vi "advanced.filter.dialog.vi"(5 "filters events":refnum<user-event>, 7 "manager_daemon":refnum<class "manager_daemon.lvclass">, 8 "filter exit event":refnum<user-event>, 9 "filtered publisher ids":i32[](array[numeric]), 10 "map":T2, 11 "pub filter event":refnum<user-event>) -> ()   [LabVIEW 2024]
uses:
  comic_manager/manager_daemon/type_defs/PublisherMap--map.ctl
  comic_manager/manager_daemon/type_defs/PublisherData--cluster.ctl
  selection_dropdown/Typedefs/Selection Dropdown--cluster.ctl
  comic_manager/manager_daemon/manager_daemon.lvclass
  typedefs/filters--cluster.ctl
  selection_dropdown/selection_dropdown.lvclass/selection_dropdown.ctl
  selection_dropdown/selection_dropdown.lvclass
  <vilib>/addons/_JKI Toolkits/State Machine/_JKI_lib_State_Machine.llb/Select State(s)_err__jki_lib_state_machine.vi
  <vilib>/addons/_JKI Toolkits/State Machine/_JKI_lib_State_Machine.llb/Periodic Trigger__ogtk__JKI-SM__jki_lib_state_machine.vi
panel:
  in  "Apply Filters":enum32{"AND", "OR"}(radio)=enum."OR"
  in  "concept filter":T1
  in  "storyArc filter":T1
  in  "character filter":T1
  in  "team filter":T1
  in  "select none":bool
  in  "select all":bool
  in  "clear error":bool
  in  "Exit":bool
  out "error out":errorcluster
  in  "pub listbox":i32(listbox)
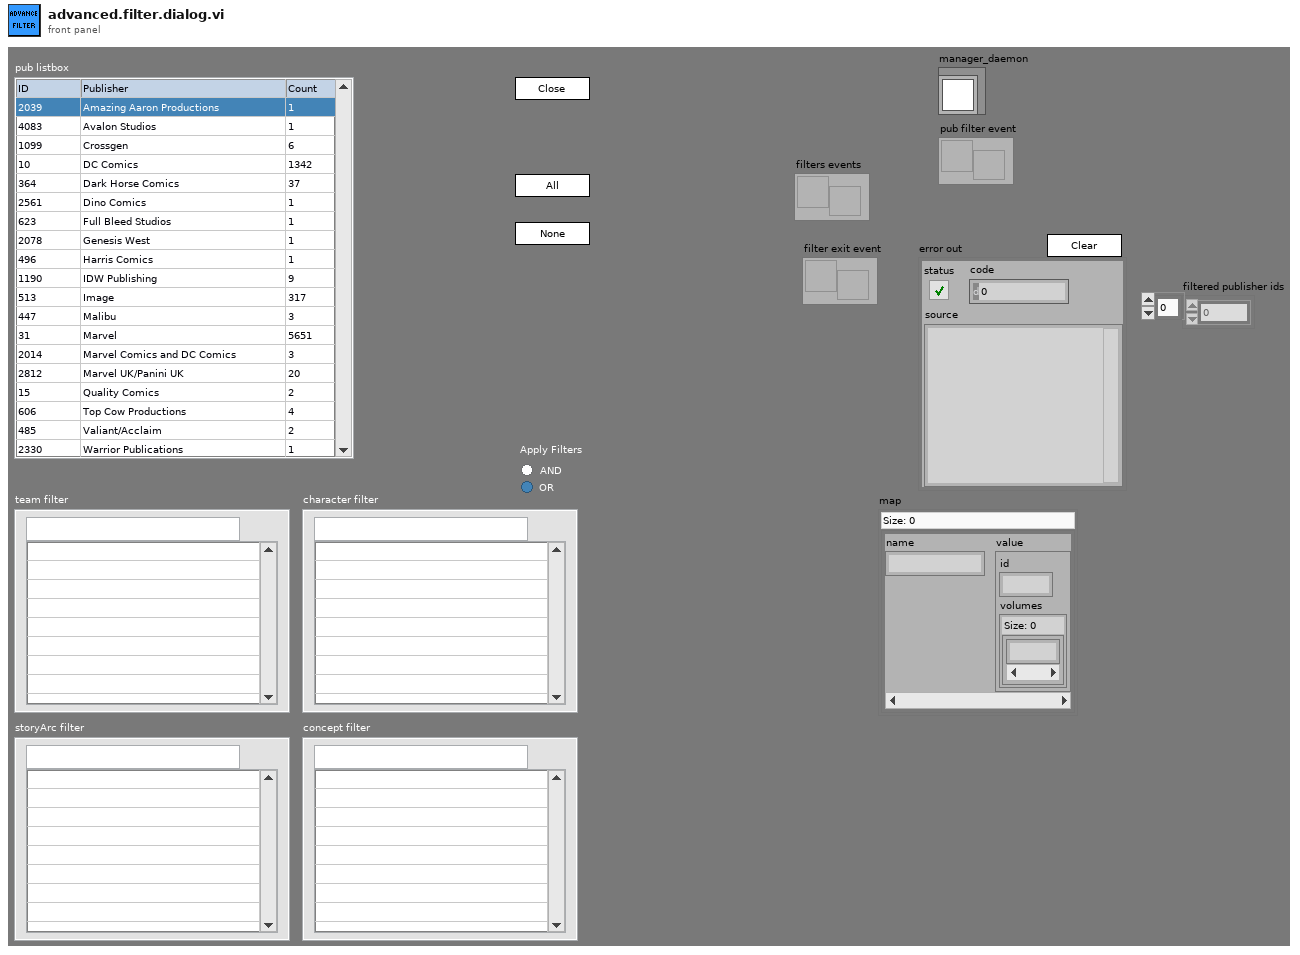
[diagram p1: front panel]
types:
  T1 = typedef "selection_dropdown.lvclass/Selection Dropdown--cluster.ctl" = cluster{"available":i32, "list":i32, "cancel":bool, "selection":string}
  T2 = typedef "manager_daemon.lvclass/PublisherMap--map.ctl" = map{string, T3}
  T3 = typedef "manager_daemon.lvclass/PublisherData--cluster.ctl" = cluster{"id":i32, "volumes":set{i32}}
  T4 = enum32{"Invalid", "Standard", "Closed", "Hidden", "Minimized", "Maximized"}
  T5 = enum32{"invalid app kind", "Development System", "Run Time System", "Student Edition", "Embedded LabVIEW", "Evaluation", "Custom"}
  T6 = typedef "filters--cluster.ctl" = cluster{"team filter":string[], "story filter":string[], "char filter":string[], "concept filter":string[], "Apply Filters":enum32{"AND", "OR"}}
  T7 = cluster{"Core":cluster{"Current VI Reference":refnum<vi>, "Close Panel on Exit?":bool}, "pub ids":i32[], "pub symbols":i32[], "pub filter event":refnum<user-event>, "filters":cluster{"team filter":refnum<class "selection_dropdown.lvclass">, "story filter":refnum<class "selection_dropdown.lvclass">, "char filter":refnum<class "selection_dropdown.lvclass">, "concept filter":refnum<class "selection_dropdown.lvclass">}, "manager_daemon":refnum<class "manager_daemon.lvclass">, "filters events":refnum<user-event>, "filter exit event":refnum<user-event>}
  T8 = cluster{"team filter":refnum<class "selection_dropdown.lvclass">, "story filter":refnum<class "selection_dropdown.lvclass">, "char filter":refnum<class "selection_dropdown.lvclass">, "concept filter":refnum<class "selection_dropdown.lvclass">}
  T9 = cluster{"Current VI Reference":refnum<vi>, "Close Panel on Exit?":bool}
  T10 = cluster{"team filter event":refnum<user-event>, "story filter event":refnum<user-event>, "char filter event":refnum<user-event>, "concept filter event":refnum<user-event>}
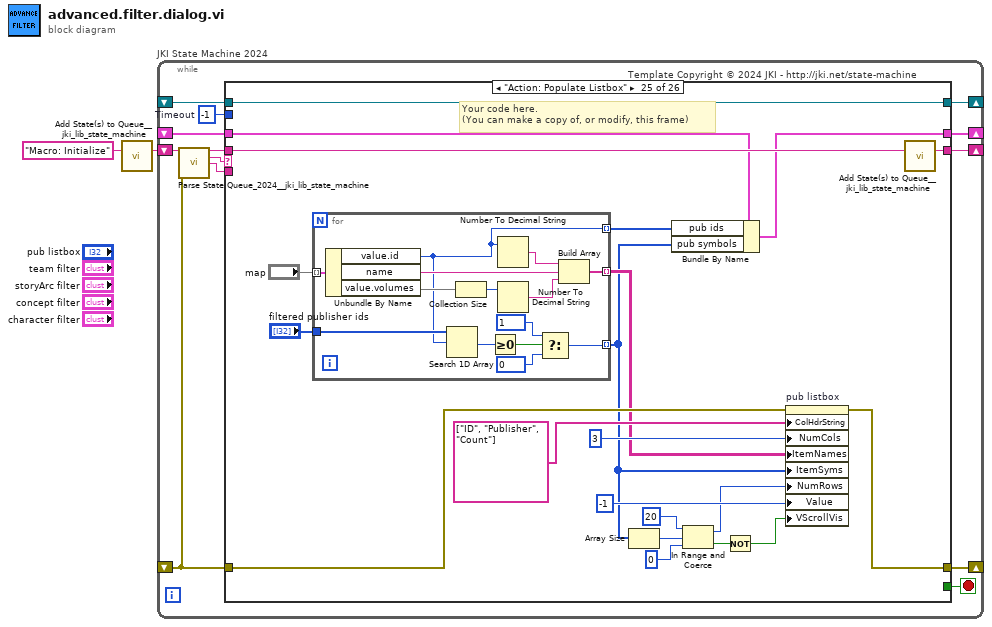
[diagram p0: block diagram]
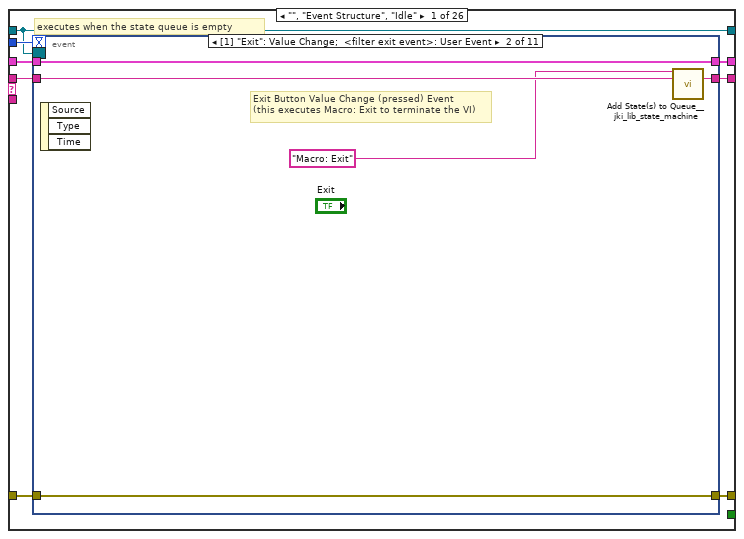
[diagram p2: hidden frame]
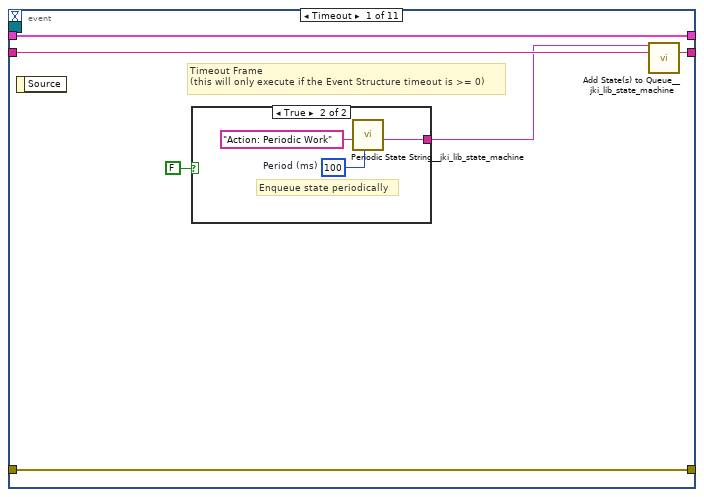
[diagram p3: hidden frame]
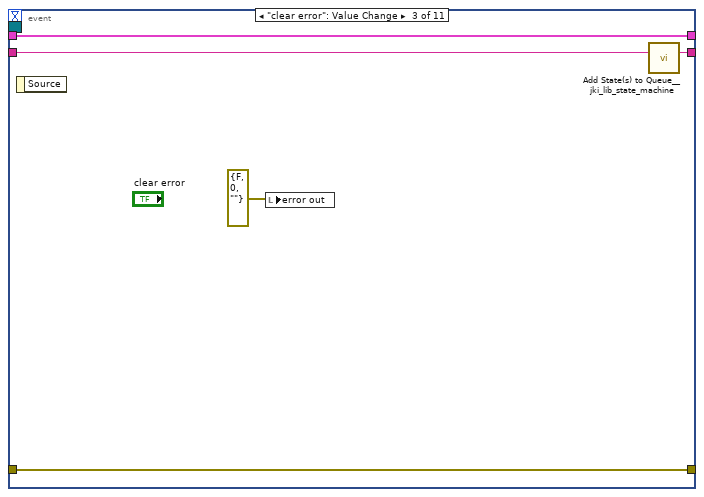
[diagram p5: hidden frame]
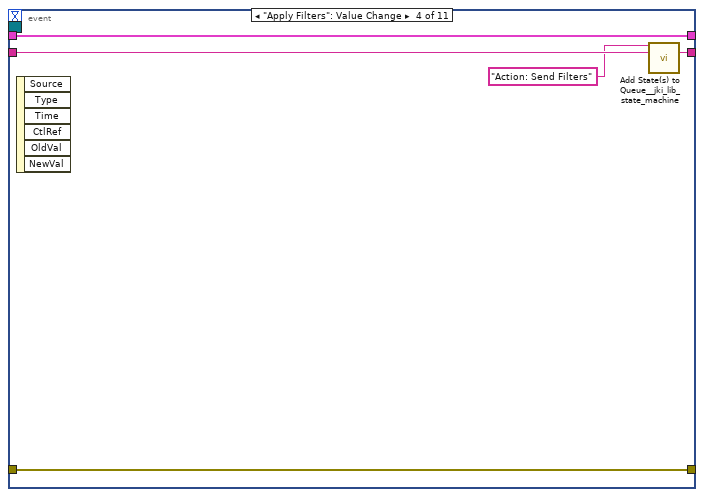
[diagram p6: hidden frame]
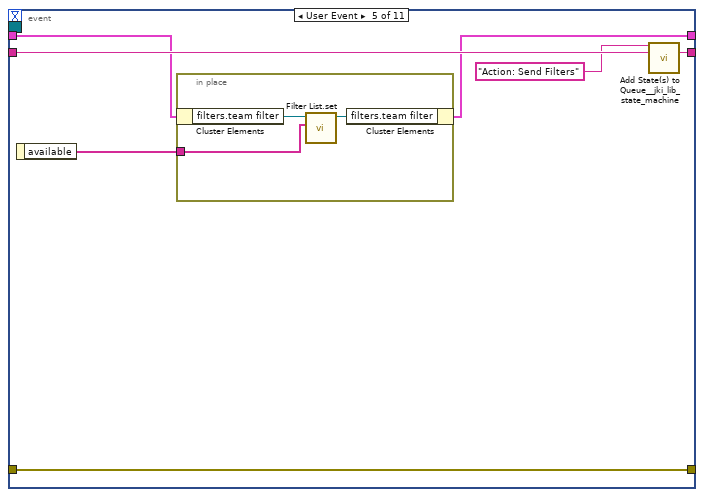
[diagram p7: hidden frame]
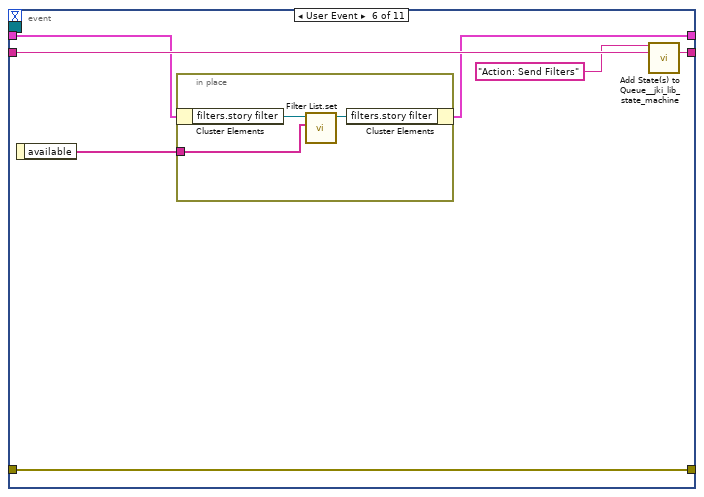
[diagram p8: hidden frame]
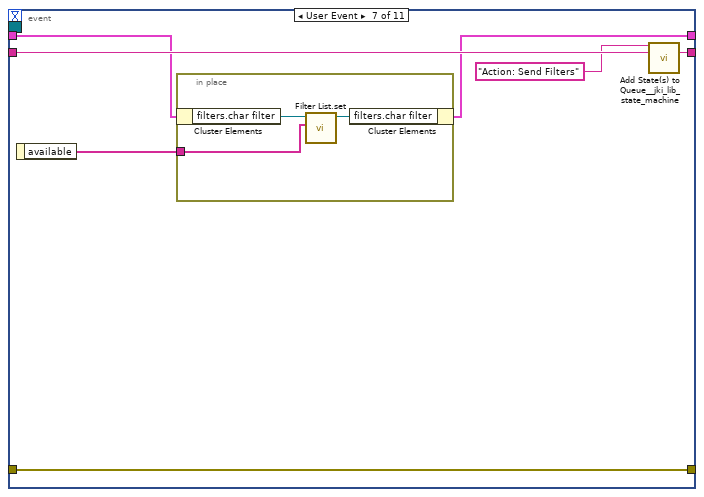
[diagram p9: hidden frame]
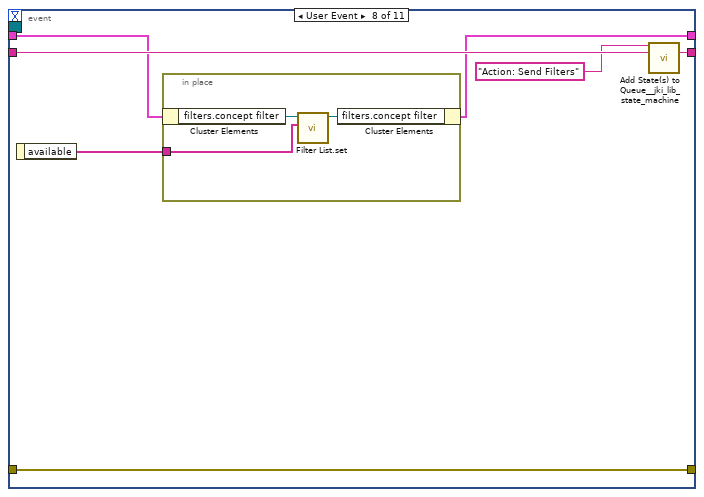
[diagram p10: hidden frame]
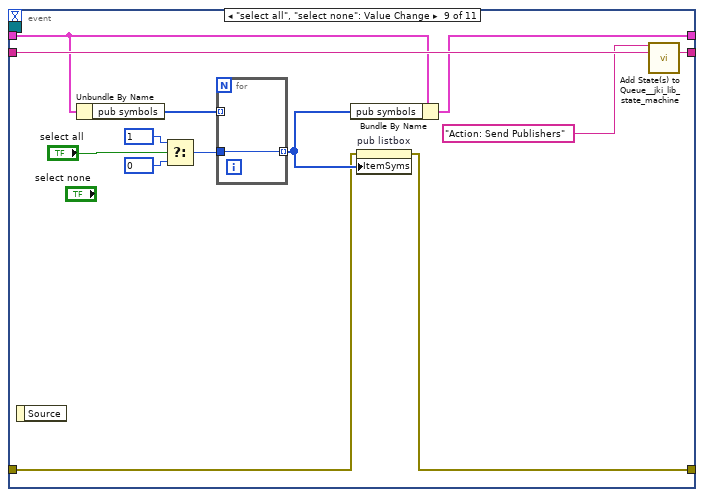
[diagram p11: hidden frame]
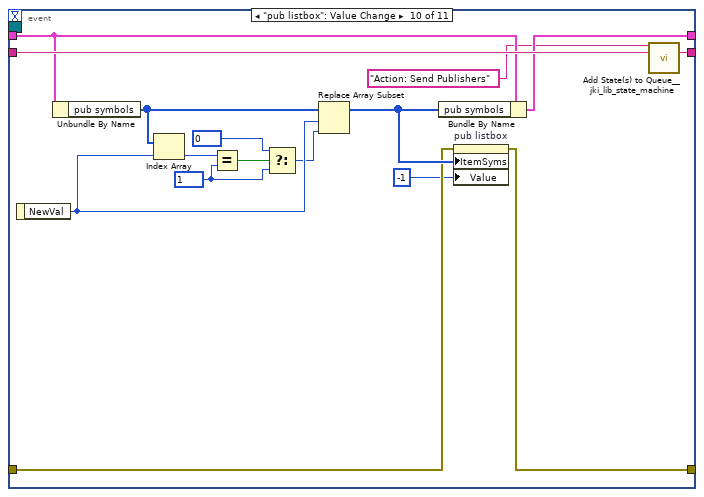
[diagram p12: hidden frame]
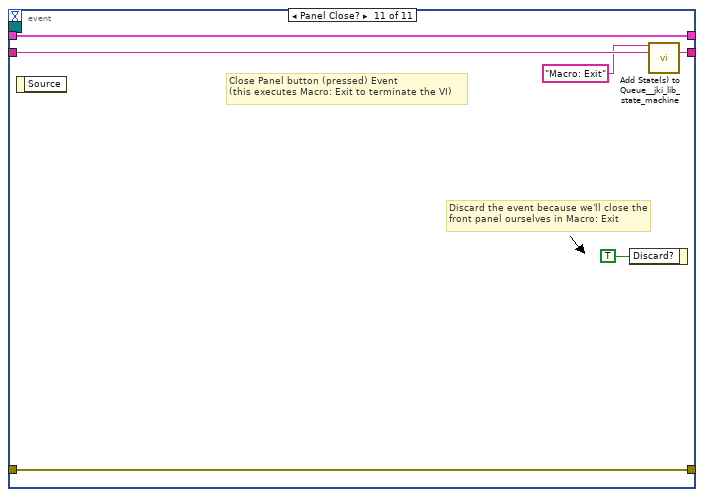
[diagram p13: hidden frame]
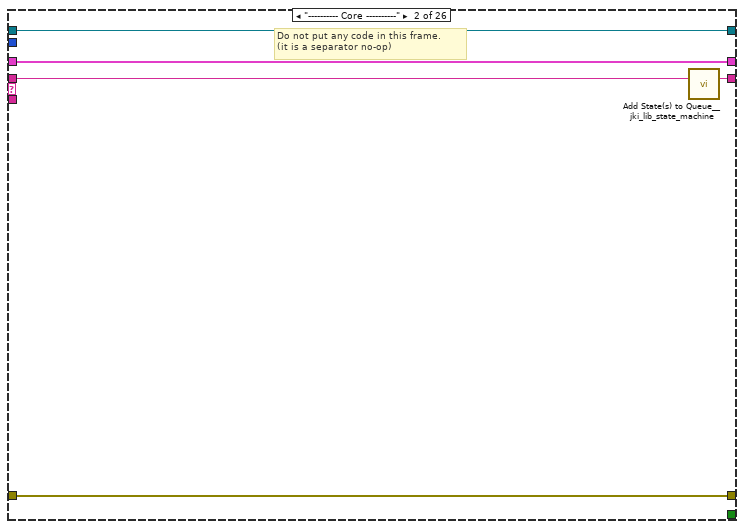
[diagram p14: hidden frame]
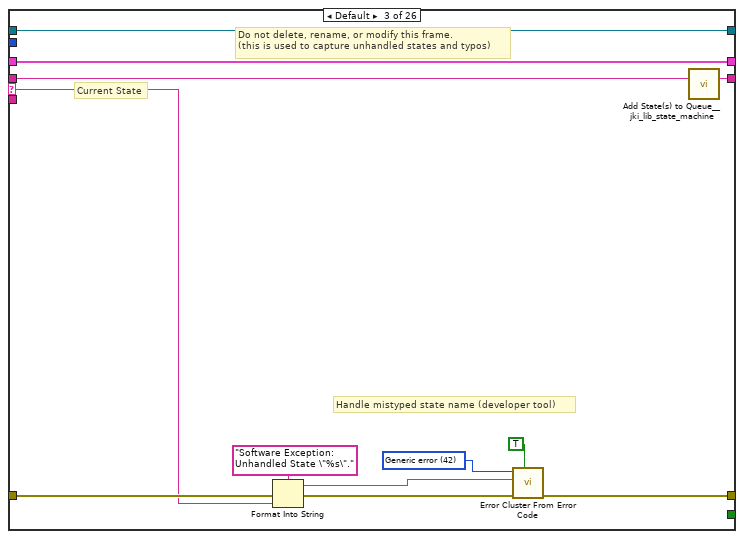
[diagram p15: hidden frame]
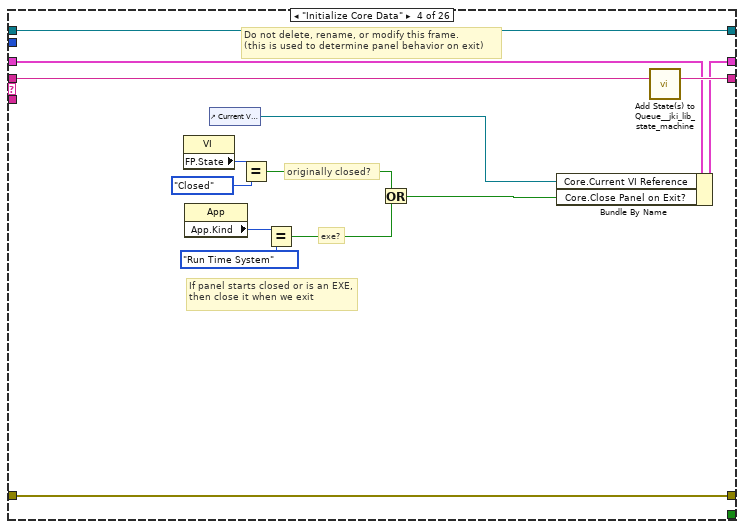
[diagram p16: hidden frame]
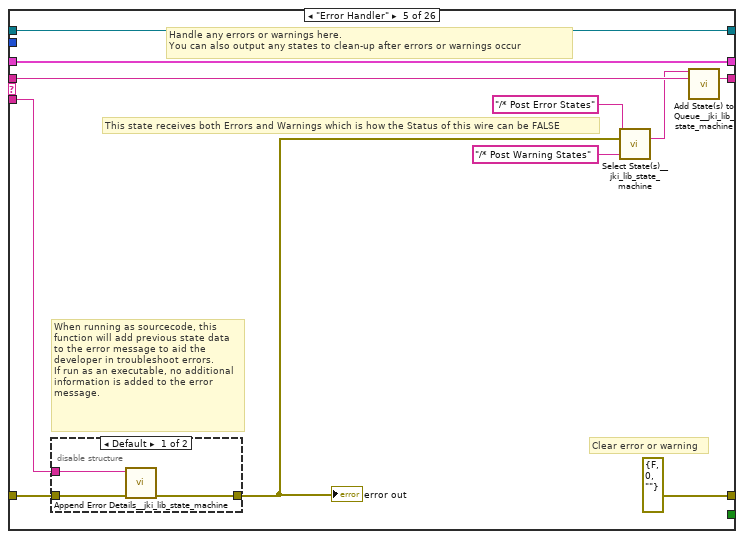
[diagram p17: hidden frame]
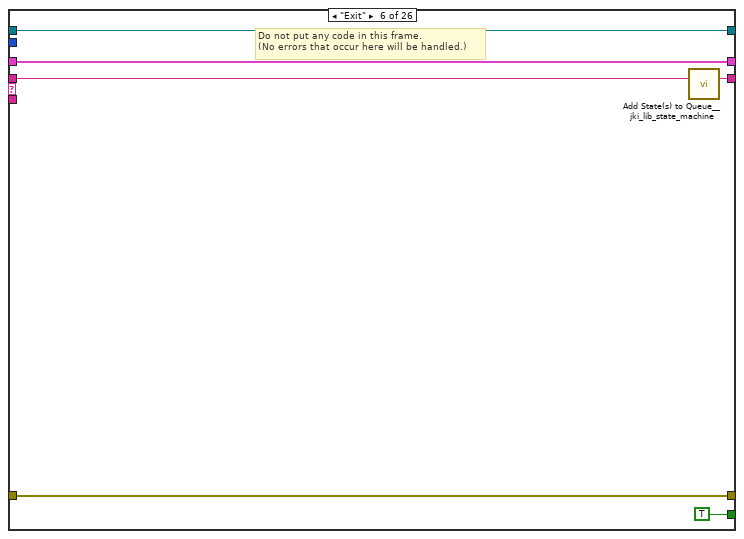
[diagram p19: hidden frame]
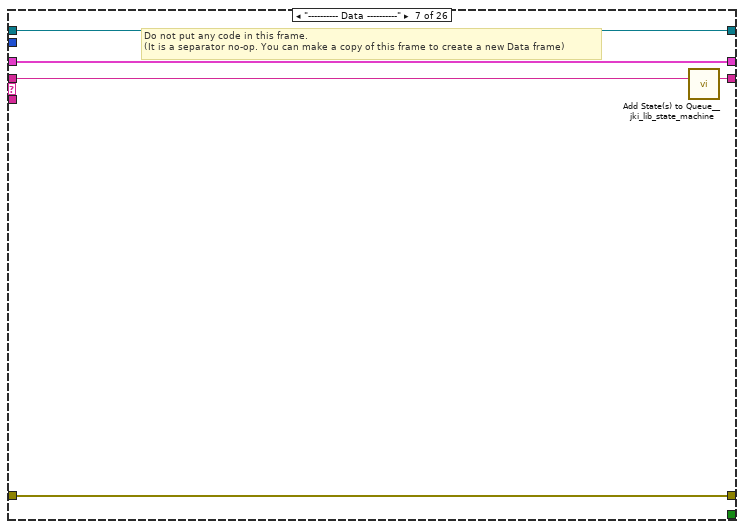
[diagram p20: hidden frame]
diagram:
  n1 = call <vilib>:"Add State(s) to Queue__jki_lib_state_machine.vi"("State(s) in (\"\")"="Macro: Initialize") -> ("States Out"=w2:string)  [unwired: 14 in]
  n2 = while "JKI State Machine 2024" {
    shift-right: [w8] -> _
    shift-left: _ -> [w7]
    shift-right: [w11] -> _
    shift-left: _ -> [w5]
    shift-right: [w10] -> _
    shift-left: w2 -> [w12]
    shift-right: [w4] -> _
    shift-left: _ -> [w3]
    stop <- w9 stop-if-true
    w6 = -1  # Timeout
    # "Template Copyright © 2024 JKI - http://jki.net/state-machine"
    n3 = call <vilib>:"Parse State Queue_2024__jki_lib_state_machine.vi"("State Queue"=w12, "Error In (no error)"=w5) -> ("Remaining States"=w14:string, "Current State"=w15:string, "Arguments"=w13:string)  [unwired: 11 in]
    n4 = case shown="\"Action: Populate Listbox\"" w15 {
      selector: w15 -> [_ _ w130 _ _ _ _ _ _ _ _ _ _ _ _ _ _ _ _ _ _ _ _ _ _ _]
      tunnel: w14 -> [w23 w128 w134 w154 w165 w175 w180 w198 w219 w224 w241 w247 w252 w257 w262 w269 w281 w351 w357 w367 w372 w390 w397 w430 w457 w481]
      tunnel: w13 -> [_ _ _ _ w160 _ _ _ _ _ _ _ _ _ _ w264 w275 _ _ _ _ _ _ _ _ _]
      tunnel: w7 -> [w21 w125 w132 w147 w162 w173 w177 _ w216 w221 w238 w245 w249 w255 w260 w267 w277 w348 w354 w365 w369 w387 w394 w427 w450 w479]
      tunnel: [w20 w126 w136 w151 errorcluster {"status"=FALSE, "code"=0, "source"=""} ("error out") w172 w178 w195 w204 w222 w239 w242 w250 w254 w259 w265 w278 w349 w355 w362 w370 w376 w391 w408 w451 w474] -> w11
      tunnel: w5 -> [w17 w126 w135 w151 w161 w172 w178 w195 w205 w222 w233 w243 w250 w254 w259 w266 w279 w349 w355 w362 w370 w377 w392 w414 w452 w475]
      tunnel: [w22 w127 w133 w153 w164 w174 w179 w197 w218 w223 w240 w246 w251 w256 w261 w268 w280 w350 w356 w366 w371 w389 w396 w429 w456 w480] -> w10
      tunnel: [_ _ _ _ _ TRUE _ _ _ _ _ _ _ _ _ _ _ _ _ _ _ _ _ _ _ _] -> w9
      tunnel: [w19 w125 w132 w152 w162 w173 w177 w196 w216 w221 w238 w245 w249 w255 w260 w267 w277 w348 w354 w365 w369 w387 w393 w404 w449 w479] -> w8
      tunnel: w6 -> [w18 _ _ _ _ _ _ _ _ _ _ _ _ _ _ _ _ _ _ _ _ _ _ _ _ _]
      tunnel: [w16 w124 w129 w141 w155 w170 w176 w184 w215 w220 w225 w244 w248 w253 w258 w263 w274 w347 w352 w358 w368 w388 w395 w428 w437 w472] -> w4
      tunnel: w3 -> [w16 w124 w129 w141 w155 w170 w176 w184 w215 w220 _ w244 w248 w253 w258 w263 w274 w347 w352 w358 w368 w388 w395 w428 w437 w472]
      frame "", "Event Structure", "Idle" {
        # "executes when the state queue is empty"
        n5 = event shown="[1] \"Exit\": Value Change;  <filter exit event>: User Event" {
          selector: w16 -> [_ _ _ _ _ _ _ _ _ _ _]
          dyn-events: _ -> [_ _ _ _ _ _ _ _ _ _ _]
          timeout: w18 -> [_ _ _ _ _ _ _ _ _ _ _]
          tunnel: w23 -> [w29 w37 w42 w47 w54 w64 w74 w84 w100 w117 w123]
          tunnel: [w28 w36 w41 w46 w53 w63 w73 w83 w99 w116 w122] -> w22
          tunnel: w21 -> [w26 w34 w39 w44 w50 w60 w70 w80 w93 w107 w120]
          tunnel: [w27 w33 w40 w45 w52 w62 w72 w82 w89 w104 w121] -> w20
          tunnel: w17 -> [w27 w33 w40 w45 w52 w62 w72 w82 w90 w105 w121]
          tunnel: [w26 w34 w39 w44 w49 w59 w69 w79 w92 w108 w120] -> w19
          event Timeout {
            # "Timeout Frame\n(this will only execute if the Event Structure timeout is >= 0)"
            n6 = event-data() -> ()  [unwired: 1 in, 1 out]
            n7 = case shown="True" FALSE {
              tunnel: [_ w32] -> w25
              frame False {
              }
              frame True {
                w30 = u32 100  # Period (ms)
                # "Enqueue state periodically"
                n8 = call <vilib>:"Periodic State String__jki_lib_state_machine.vi"("Period (ms)"=w30, "State"="Action: Periodic Work") -> ("State Out"=w32:string)  [unwired: 9 in]
              }
            }
            n9 = call <vilib>:"Add State(s) to Queue__jki_lib_state_machine.vi"("State(s) in Front (\"\")"=w25, "State(s) in (\"\")"=w29) -> ("States Out"=w28:string)  [unwired: 13 in]
          }
          event "Exit": Value Change; User Event {
            # "Exit Button Value Change (pressed) Event\n(this executes Macro: Exit to terminate the VI)"
            n10 = event-data() -> ()  [unwired: 1 in, 3 out]
            n11 = call <vilib>:"Add State(s) to Queue__jki_lib_state_machine.vi"("State(s) in Front (\"\")"="Macro: Exit", "State(s) in (\"\")"=w37) -> ("States Out"=w36:string)  [unwired: 13 in]
          }
          event "clear error": Value Change {
            n12 = event-data() -> ()  [unwired: 1 in, 1 out]
            n13 = local write "error out"(errorcluster {"status"=FALSE, "code"=0, "source"=""} ("error out")) -> ()
            n14 = call <vilib>:"Add State(s) to Queue__jki_lib_state_machine.vi"("State(s) in (\"\")"=w42) -> ("States Out"=w41:string)  [unwired: 14 in]
          }
          event "Apply Filters": Value Change {
            n15 = event-data() -> ()  [unwired: 1 in, 6 out]
            n16 = call <vilib>:"Add State(s) to Queue__jki_lib_state_machine.vi"("State(s) in Front (\"\")"="Action: Send Filters" ("State(s) in Front (\"\")"), "State(s) in (\"\")"=w47) -> ("States Out"=w46:string)  [unwired: 13 in]
          }
          event User Event {
            n17 = event-data() -> ("available"=w51:string[])  [unwired: 1 in]
            n18 = in-place {
              in-place-border: w51 -> [w55]
              n19 = in-place-cluster #1(w50) -> ("filters.team filter"=w57:refnum<class "selection_dropdown.lvclass">)
              n20 = call "Filter List.set.vi"("filter list"=w55, "selection_dropdown in"=w57) -> ("selection_dropdown out"=w56:refnum<class "selection_dropdown.lvclass">)  [unwired: 9 in]
              n21 = in-place-cluster #1("filters.team filter"=w56) -> (w49:T7)
            }
            n22 = call <vilib>:"Add State(s) to Queue__jki_lib_state_machine.vi"("State(s) in Front (\"\")"="Action: Send Filters" ("State(s) in Front (\"\")"), "State(s) in (\"\")"=w54) -> ("States Out"=w53:string)  [unwired: 13 in]
          }
          event User Event {
            n23 = event-data() -> ("available"=w61:string[])  [unwired: 1 in]
            n24 = in-place {
              in-place-border: w61 -> [w65]
              n25 = in-place-cluster #2(w60) -> ("filters.story filter"=w67:refnum<class "selection_dropdown.lvclass">)
              n26 = call "Filter List.set.vi"("filter list"=w65, "selection_dropdown in"=w67) -> ("selection_dropdown out"=w66:refnum<class "selection_dropdown.lvclass">)  [unwired: 9 in]
              n27 = in-place-cluster #2("filters.story filter"=w66) -> (w59:T7)
            }
            n28 = call <vilib>:"Add State(s) to Queue__jki_lib_state_machine.vi"("State(s) in Front (\"\")"="Action: Send Filters" ("State(s) in Front (\"\")"), "State(s) in (\"\")"=w64) -> ("States Out"=w63:string)  [unwired: 13 in]
          }
          event User Event {
            n29 = event-data() -> ("available"=w71:string[])  [unwired: 1 in]
            n30 = in-place {
              in-place-border: w71 -> [w75]
              n31 = in-place-cluster #3(w70) -> ("filters.char filter"=w77:refnum<class "selection_dropdown.lvclass">)
              n32 = call "Filter List.set.vi"("filter list"=w75, "selection_dropdown in"=w77) -> ("selection_dropdown out"=w76:refnum<class "selection_dropdown.lvclass">)  [unwired: 9 in]
              n33 = in-place-cluster #3("filters.char filter"=w76) -> (w69:T7)
            }
            n34 = call <vilib>:"Add State(s) to Queue__jki_lib_state_machine.vi"("State(s) in Front (\"\")"="Action: Send Filters" ("State(s) in Front (\"\")"), "State(s) in (\"\")"=w74) -> ("States Out"=w73:string)  [unwired: 13 in]
          }
          event User Event {
            n35 = event-data() -> ("available"=w81:string[])  [unwired: 1 in]
            n36 = in-place {
              in-place-border: w81 -> [w85]
              n37 = in-place-cluster #4(w80) -> ("filters.concept filter"=w87:refnum<class "selection_dropdown.lvclass">)
              n38 = call "Filter List.set.vi"("filter list"=w85, "selection_dropdown in"=w87) -> ("selection_dropdown out"=w86:refnum<class "selection_dropdown.lvclass">)  [unwired: 9 in]
              n39 = in-place-cluster #4("filters.concept filter"=w86) -> (w79:T7)
            }
            n40 = call <vilib>:"Add State(s) to Queue__jki_lib_state_machine.vi"("State(s) in Front (\"\")"="Action: Send Filters" ("State(s) in Front (\"\")"), "State(s) in (\"\")"=w84) -> ("States Out"=w83:string)  [unwired: 13 in]
          }
          event "select all", "select none": Value Change {
            n41 = event-data() -> ()  [unwired: 1 in, 1 out]
            n42 = Unbundle By Name(w93) -> ("pub symbols"=w98:i32[])
            n43 = Select(t=1, s="select all", f=0) -> (s? t:f=w94:i32)
            n44 = for {
              tunnel: w98 -> [_] mode=indexing
              tunnel: w94 -> [w101]
              tunnel: [w101] -> w91 mode=indexing
            }
            n45 = Bundle By Name(cluster=w93, "pub symbols"=w91) -> (w92:T7)
            n46 = property on="pub listbox" class="MCListbox (strict)"(error in=w90, "ItemSyms"=w91) -> (error out=w89:errorcluster)  [unwired: 1 in, 1 out]
            n47 = call <vilib>:"Add State(s) to Queue__jki_lib_state_machine.vi"("State(s) in Front (\"\")"="Action: Send Publishers" ("State(s) in Front (\"\")"), "State(s) in (\"\")"=w100) -> ("States Out"=w99:string)  [unwired: 13 in]
          }
          event "pub listbox": Value Change {
            w113 = 1
            n48 = event-data() -> ("NewVal"=w110:i32)  [unwired: 1 in]
            n49 = Unbundle By Name(w107) -> ("pub symbols"=w111:i32[])
            n50 = Index Array(array=w111, index=w110) -> (element=w115:i32)
            n51 = Equal?(x=w115, y=w113) -> (x = y?=w114:bool)
            n52 = Select(t=0, s=w114, f=w113) -> (s? t:f=w109:i32)
            n53 = Replace Array Subset(array=w111, new element=w109, index=w110) -> (w106:i32[])
            n54 = Bundle By Name(cluster=w107, "pub symbols"=w106) -> (w108:T7)
            n55 = property on="pub listbox" class="MCListbox (strict)"(error in=w105, "ItemSyms"=w106, "Value"=-1 ("Publishers")) -> (error out=w104:errorcluster)  [unwired: 1 in, 1 out]
            n56 = call <vilib>:"Add State(s) to Queue__jki_lib_state_machine.vi"("State(s) in Front (\"\")"="Action: Send Publishers" ("State(s) in Front (\"\")"), "State(s) in (\"\")"=w117) -> ("States Out"=w116:string)  [unwired: 13 in]
          }
          event Panel Close? {
            # "Discard the event because we'll close the front panel ourselves in Macro: Exit"
            # "Close Panel button (pressed) Event\n(this executes Macro: Exit to terminate the VI)"
            n57 = event-data() -> ()  [unwired: 1 in, 1 out]
            n58 = event-data("Discard?"=TRUE) -> ()  [unwired: 1 in, 1 out]
            n59 = call <vilib>:"Add State(s) to Queue__jki_lib_state_machine.vi"("State(s) in Front (\"\")"="Macro: Exit", "State(s) in (\"\")"=w123) -> ("States Out"=w122:string)  [unwired: 13 in]
          }
        }
      }
      frame "---------- Core ----------" {
        # "Do not put any code in this frame.\n(it is a separator no-op)"
        n60 = call <vilib>:"Add State(s) to Queue__jki_lib_state_machine.vi"("State(s) in (\"\")"=w128) -> ("States Out"=w127:string)  [unwired: 14 in]
      }
      frame Default {
        w139 = 42 items=["No error", "Argument error", "Memory is full", "Out of zone", "End of file", "File already open", "Generic file I/O error", "File not found", "File permission error", "Disk is full", "Duplicate path", "Too many files open", "System feature not enabled", "Resource file not found", "Cannot add resource", "Resource not found", "Image not found", "Image memory error", "Pen does not exist", "Config type invalid", "Config token not found", "Config parse error", "Config memory error", "Bad external code format", "Bad external code offset", "External code not present", "Null window", "Destroy window error", "Null menu", "Print aborted", "Bad print record", "Print driver error", "Windows error during printing", "Memory error during printing", "Print dialog error", "Generic print error", "Invalid device refnum", "Device not found", "Device parameter error", "Device unit error", "Cannot open device", "Device call aborted", "Generic error", "Cancelled by user", "Object ID too low", "Object ID too high", "Object not in heap", "Unknown heap", "Unknown object (invalid DefProc)", "Unknown object (DefProc not in table)", "Message out of range", "Invalid (null) method", "Unknown message", "Manager call not supported", "Bad address", "Network operation in progress", "Network operation timed out", "Connection is busy", "Network attribute not supported", "Network error", "Address in use", "System out of memory", "Connection aborted", "Connection refused", "Not connected", "Already connected", "Connection closed", "Initialization error (interapplication manager)", "Bad occurrence", "Wait on unbound occurrence handler", "Occurrence queue overflow", "Datalog type conflict", "Unused", "Unrecognized type (interapplication manager)", "Memory corrupt", "Failed to make temporary DLL", "Old CIN version", "Drag socket not found", "Failed to load drop-object", "Failed to register OLE object", "Failed to release OLE object", "Format specifier type mismatch", "Unknown format specifier", "Too few format specifiers", "Too many format specifiers", "Scan failed", "Newer CIN version", "Error converting to variant", "Runtime menu error", "Password tampered", "Variant attribute not found", "Incompatible variant data type", "Event data is not available", "Event Store is not present", "Occurrence is not found", "Event Queue is not created", "Event info is not available", "Refnum passed is NULL", "Error retrieving Class GUID", "Error retrieving CoClass GUID", "Error retrieving TypeLib GUID.", "Bad built application magic bytes.", "Specific driver is different from the specific driver associated with the Logical Name.", "There is no session opened to the class driver.", "Max Error", "MAX - Error with config objects", "MAX - Error loading configuration", "MAX - Group not supported"]
        # "Current State"
        # "Do not delete, rename, or modify this frame.\n(this is used to capture unhandled states and typos)"
        # "Handle mistyped state name (developer tool)"
        n61 = Format Into String(format string="Software Exception: Unhandled State \"%s\"." ("message"), error in=w135, w130) -> (resulting string=w138:string, error out=w137:errorcluster)  [unwired: 1 in]
        n62 = call <vilib>:"Error Cluster From Error Code.vi"("show call chain? (False)"=TRUE, "error in (no error)"=w137, "error message (\"\")"=w138, "error code (0)"=w139) -> ("error out"=w136:errorcluster)  [unwired: 5 in]
        n63 = call <vilib>:"Add State(s) to Queue__jki_lib_state_machine.vi"("State(s) in (\"\")"=w134) -> ("States Out"=w133:string)  [unwired: 14 in]
      }
      frame "Initialize Core Data" {
        # "Do not delete, rename, or modify this frame.\n(this is used to determine panel behavior on exit)"
        # "originally closed?"
        # "exe?"
        # "If panel starts closed or is an EXE, then close it when we exit"
        n64 = property class="VI"() -> ("FP.State"=w144:T4)  [unwired: 2 in, 2 out]
        n65 = property class="App"() -> ("App.Kind"=w150:T5)  [unwired: 2 in, 2 out]
        n66 = control-ref of="Current VI Reference"() -> (w145:refnum<vi>)
        n67 = Equal?(x=w144, y=T4."Closed" ("Front Panel Window:State")) -> (x = y?=w142:bool)
        n68 = Equal?(x=w150, y=T5."Run Time System" ("Application:Kind")) -> (x = y?=w148:bool)
        n69 = Or(x=w142, y=w148) -> (x .or. y?=w146:bool)
        n70 = Bundle By Name(cluster=w147, "Core.Current VI Reference"=w145, "Core.Close Panel on Exit?"=w146) -> (w152:T7)
        n71 = call <vilib>:"Add State(s) to Queue__jki_lib_state_machine.vi"("State(s) in (\"\")"=w154) -> ("States Out"=w153:string)  [unwired: 14 in]
      }
      frame "Error Handler" {
        # "When running as sourcecode, this function will add previous state data to the error message to aid the developer in troubleshoot errors.\nIf run as an executable, no additional information is added to the error message."
        # "This state receives both Errors and Warnings which is how the Status of this wire can be FALSE"
        # "Handle any errors or warnings here.\nYou can also output any states to clean-up after errors or warnings occur"
        # "Clear error or warning"
        n72 = disable-structure shown="Default" {
          disable-tunnel: w161 -> [w168 w169]
          disable-tunnel: w160 -> [w167 _]
          disable-tunnel: [w166 w169] -> w156
          frame condition #0 (active) {
            n73 = call <vilib>:"Append Error Details__jki_lib_state_machine.vi"("error in (no error)"=w168, "Previous State and Argument(s)"=w167) -> ("error out"=w166:errorcluster)  [unwired: 9 in]
          }
          frame condition #1 {
          }
        }
        "error out" <- w156
        n74 = call-poly <vilib>:"Select State(s)__jki_lib_state_machine.vi"("State(s) if True (\"\")"="/* Post Error States", "Select"=w156, "State(s) if False (\"\")"="/* Post Warning States") -> ("States Out"=w158:string)  [unwired: 12 in]
        n75 = call <vilib>:"Add State(s) to Queue__jki_lib_state_machine.vi"("State(s) in Front (\"\")"=w158, "State(s) in (\"\")"=w165) -> ("States Out"=w164:string)  [unwired: 13 in]
      }
      frame "Exit" {
        # "Do not put any code in this frame.\n(No errors that occur here will be handled.)"
        n76 = call <vilib>:"Add State(s) to Queue__jki_lib_state_machine.vi"("State(s) in (\"\")"=w175) -> ("States Out"=w174:string)  [unwired: 14 in]
      }
      frame "---------- Data ----------" {
        # "Do not put any code in this frame.\n(It is a separator no-op. You can make a copy of this frame to create a new Data frame)"
        n77 = call <vilib>:"Add State(s) to Queue__jki_lib_state_machine.vi"("State(s) in (\"\")"=w180) -> ("States Out"=w179:string)  [unwired: 14 in]
      }
      frame "Data: Initialize" {
        w186 = T8 {"team filter"=refnum, "story filter"=refnum, "char filter"=refnum, "concept filter"=refnum}  # filters
        w187 = refnum<class "selection_dropdown.lvclass"> refnum  # concept filter
        w189 = refnum<class "selection_dropdown.lvclass"> refnum  # story filter
        w188 = refnum<class "selection_dropdown.lvclass"> refnum  # char filter
        w190 = refnum<class "selection_dropdown.lvclass"> refnum  # team filter
        w192 = i32[] []  # pub ids
        w193 = i32[] []  # pub symbols
        w194 = T9 {"Current VI Reference"=refnum, "Close Panel on Exit?"=FALSE}  # Core
        # "Initialize the shift-register data, here.\n(data names are defined by what you wire into the bundle function)"
        n78 = Bundle(cluster=w186, "team filter"=w190, "story filter"=w189, "char filter"=w188, "concept filter"=w187) -> (w185:T8)
        n79 = Bundle("Core"=w194, "pub ids"=w192, "pub symbols"=w193, "pub filter event"="pub filter event", "filters"=w185, "manager_daemon"="manager_daemon", "filters events"="filters events", "filter exit event"="filter exit event") -> (w196:T7)  [unwired: 1 in]
        n80 = call <vilib>:"Add State(s) to Queue__jki_lib_state_machine.vi"("State(s) in (\"\")"=w198) -> ("States Out"=w197:string)  [unwired: 14 in]
      }
      frame "Data: Cleanup" {
        # "Cleanup any data and references, here.\n(this is called automatically, by the Macro: Exit)"
        n81 = Unbundle By Name(w216) -> ("Core.Current VI Reference"=w217:refnum<vi>, "filters.team filter"=w214:refnum<class "selection_dropdown.lvclass">, "filters.story filter"=w213:refnum<class "selection_dropdown.lvclass">, "filters.char filter"=w212:refnum<class "selection_dropdown.lvclass">, "filters.concept filter"=w211:refnum<class "selection_dropdown.lvclass">, "filter exit event"=w202:refnum<user-event>)
        n82 = Generate User Event(user event=w202, event data cluster=TRUE ("event data")) -> (error out=w200:errorcluster)  [unwired: 2 in, 1 out]
        n83 = call "Destroy.vi"("selection_dropdown in"=w211) -> ("error out"=w210:errorcluster)  [unwired: 9 in, 1 out]
        n84 = call "Destroy.vi"("selection_dropdown in"=w212) -> ("error out"=w209:errorcluster)  [unwired: 9 in, 1 out]
        n85 = call <vilib>:"Clear Errors.vi"("error in (no error)"=w200, "specific error code to clear (0: all)"=1) -> ("error out"=w199:errorcluster)  [unwired: 4 in, 1 out]
        n86 = call "Destroy.vi"("selection_dropdown in"=w213) -> ("error out"=w208:errorcluster)  [unwired: 9 in, 1 out]
        n87 = call "Destroy.vi"("selection_dropdown in"=w214) -> ("error out"=w207:errorcluster)  [unwired: 9 in, 1 out]
        n88 = Close Reference(reference=w217) -> (error out=w206:errorcluster)  [unwired: 1 in]
        n89 = Merge Errors(w205, w206, w207, w208, w209, w210, w199) -> (w204:errorcluster)
        n90 = call <vilib>:"Add State(s) to Queue__jki_lib_state_machine.vi"("State(s) in (\"\")"=w219) -> ("States Out"=w218:string)  [unwired: 14 in]
      }
      frame "---------- Events ----------" {
        # "Do not put any code in this frame.\n(It is a separator no-op. You can make a copy of this frame to create a new UI frame)"
        n91 = call <vilib>:"Add State(s) to Queue__jki_lib_state_machine.vi"("State(s) in (\"\")"=w224) -> ("States Out"=w223:string)  [unwired: 14 in]
      }
      frame "Events: Register" {
        w227 = T10 {"team filter event"=refnum, "story filter event"=refnum, "char filter event"=refnum, "concept filter event"=refnum}  # filter events
        # "Do not put any code in this frame.\n(It is a separator no-op. You can make a copy of this frame to create a new UI frame)"
        n92 = Unbundle By Name(w238) -> ("filters.team filter"=w237:refnum<class "selection_dropdown.lvclass">, "filters.story filter"=w236:refnum<class "selection_dropdown.lvclass">, "filters.char filter"=w235:refnum<class "selection_dropdown.lvclass">, "filters.concept filter"=w234:refnum<class "selection_dropdown.lvclass">, "filter exit event"=w226:refnum<user-event>)
        n93 = call "Filter List Event.get.vi"("selection_dropdown in"=w237) -> ("filter list event"=w232:refnum<user-event>)  [unwired: 9 in, 1 out]
        n94 = call "Filter List Event.get.vi"("selection_dropdown in"=w236) -> ("filter list event"=w231:refnum<user-event>)  [unwired: 9 in, 1 out]
        n95 = call "Filter List Event.get.vi"("selection_dropdown in"=w235) -> ("filter list event"=w230:refnum<user-event>)  [unwired: 9 in, 1 out]
        n96 = call "Filter List Event.get.vi"("selection_dropdown in"=w234) -> ("filter list event"=w229:refnum<user-event>)  [unwired: 9 in, 1 out]
        n97 = Bundle(cluster=w227, "team filter event"=w232, "story filter event"=w231, "char filter event"=w230, "concept filter event"=w229) -> (w228:T10)
        n98 = register-events(error in=w233, w228, w226) -> (reference out=w225:refnum<event-registration>, error out=w239:errorcluster)  [unwired: 1 in]
        n99 = call <vilib>:"Add State(s) to Queue__jki_lib_state_machine.vi"("State(s) in (\"\")"=w241) -> ("States Out"=w240:string)  [unwired: 14 in]
      }
      frame "Events: Unregister" {
        # "Do not put any code in this frame.\n(It is a separator no-op. You can make a copy of this frame to create a new UI frame)"
        n100 = Unregister For Events(event registration refnum=w244, error in=w243) -> (error out=w242:errorcluster)
        n101 = call <vilib>:"Add State(s) to Queue__jki_lib_state_machine.vi"("State(s) in (\"\")"=w247) -> ("States Out"=w246:string)  [unwired: 14 in]
      }
      frame "---------- UI ----------" {
        # "Do not put any code in this frame.\n(It is a separator no-op. You can make a copy of this frame to create a new UI frame)"
        n102 = call <vilib>:"Add State(s) to Queue__jki_lib_state_machine.vi"("State(s) in (\"\")"=w252) -> ("States Out"=w251:string)  [unwired: 14 in]
      }
      frame "UI: Initialize" {
        # "Initialize the User Interface, here.\n(this is called automatically, by the Macro: Initialize)"
        n103 = call <vilib>:"Add State(s) to Queue__jki_lib_state_machine.vi"("State(s) in (\"\")"=w257) -> ("States Out"=w256:string)  [unwired: 14 in]
      }
      frame "UI: Uninitialize" {
        # "Cleanup the User Interface, here.\n(this is called automatically, by the Macro: Exit)"
        n104 = call <vilib>:"Add State(s) to Queue__jki_lib_state_machine.vi"("State(s) in (\"\")"=w262) -> ("States Out"=w261:string)  [unwired: 14 in]
      }
      frame "UI: Cursor Set" {
        # "Argument"
        # "Set and Unset Cursor Busy.\n(Usage: \"UI: Cursor Set >> Busy|Idle\")"
        n105 = case shown="\"Idle\", Default" w264 {
          tunnel: w266 -> [w271 w273]
          tunnel: [w270 w272] -> w265
          frame "Idle", Default {
            n106 = call <vilib>:"Unset Busy.vi"("error in (no error)"=w271) -> ("error out"=w270:errorcluster)  [unwired: 10 in]
          }
          frame "Busy" {
            n107 = call <vilib>:"Set Busy.vi"("error in (no error)"=w273) -> ("error out"=w272:errorcluster)  [unwired: 9 in, 1 out]
          }
        }
        n108 = call <vilib>:"Add State(s) to Queue__jki_lib_state_machine.vi"("State(s) in (\"\")"=w269) -> ("States Out"=w268:string)  [unwired: 14 in]
      }
      frame "UI: Front Panel State" {
        # "Argument"
        # "Set Front Panel Open or Closed\n(Usage: \"UI: Front Panel State >> Open|Close\")"
        n109 = Unbundle By Name(w277) -> ("Core.Current VI Reference"=w276:refnum<vi>)
        n110 = case shown="\"Open\", \"Standard\", Default" w275 {
          tunnel: w279 -> [w287 w302 w313 w326 w339]
          tunnel: [w289 w303 w315 w328 w341] -> w278
          tunnel: w276 -> [w288 w300 w314 w327 w340]
          frame "Open", "Standard", Default {
            w282 = T4."Standard" ("State")
            n111 = property class="VI"(reference=w288, error in=w287) -> (reference out=w285:refnum<vi>, error out=w286:errorcluster, "FP.State"=w284:T4)
            n112 = Not Equal?(x=w284, y=w282) -> (x != y?=w283:bool)
            n113 = case shown="False" w283 {
              tunnel: [w293 w295] -> w289
              tunnel: w286 -> [w292 w295]
              tunnel: w285 -> [w291 _]
              tunnel: w282 -> [w290 _]
              frame True {
                n114 = invoke class="VI" method="FP.Open"(reference=w291, error in=w292, "Activate"=TRUE, "State"=w290) -> (error out=w293:errorcluster)  [unwired: 1 in, 4 out]
              }
              frame False {
              }
            }
          }
          frame "Close", "Closed" {
            n115 = property class="VI"(reference=w300, error in=w302) -> (reference out=w299:refnum<vi>, error out=w301:errorcluster, "FP.State"=w297:T4)
            n116 = Not Equal?(x=w297, y=T4."Closed" ("Front Panel Window:State")) -> (x != y?=w296:bool)
            n117 = case shown="True" w296 {
              tunnel: [w304 w307] -> w303
              tunnel: w301 -> [w304 w306]
              tunnel: w299 -> [_ w305]
              frame False {
              }
              frame True {
                n118 = invoke class="VI" method="FP.Close"(reference=w305, error in=w306) -> (error out=w307:errorcluster)  [unwired: 1 in, 2 out]
              }
            }
          }
          frame "Hidden", "Hide" {
            w308 = T4."Hidden" ("State")
            n119 = property class="VI"(reference=w314, error in=w313) -> (reference out=w311:refnum<vi>, error out=w312:errorcluster, "FP.State"=w310:T4)
            n120 = Not Equal?(x=w310, y=w308) -> (x != y?=w309:bool)
            n121 = case shown="True" w309 {
              tunnel: [w319 w320] -> w315
              tunnel: w312 -> [w318 w320]
              tunnel: w311 -> [w317 _]
              tunnel: w308 -> [w316 _]
              frame True {
                n122 = invoke class="VI" method="FP.Open"(reference=w317, error in=w318, "State"=w316) -> (error out=w319:errorcluster)  [unwired: 2 in, 4 out]
              }
              frame False {
              }
            }
          }
          frame "Minimize", "Minimized" {
            w321 = T4."Minimized" ("State")
            n123 = property class="VI"(reference=w327, error in=w326) -> (reference out=w324:refnum<vi>, error out=w325:errorcluster, "FP.State"=w323:T4)
            n124 = Not Equal?(x=w323, y=w321) -> (x != y?=w322:bool)
            n125 = case shown="True" w322 {
              tunnel: [w332 w333] -> w328
              tunnel: w325 -> [w331 w333]
              tunnel: w324 -> [w330 _]
              tunnel: w321 -> [w329 _]
              frame True {
                n126 = invoke class="VI" method="FP.Open"(reference=w330, error in=w331, "State"=w329) -> (error out=w332:errorcluster)  [unwired: 2 in, 4 out]
              }
              frame False {
              }
            }
          }
          frame "Maximize", "Maximized" {
            w334 = T4."Maximized" ("State")
            n127 = property class="VI"(reference=w340, error in=w339) -> (reference out=w337:refnum<vi>, error out=w338:errorcluster, "FP.State"=w336:T4)
            n128 = Not Equal?(x=w336, y=w334) -> (x != y?=w335:bool)
            n129 = case shown="True" w335 {
              tunnel: [w345 w346] -> w341
              tunnel: w338 -> [w344 w346]
              tunnel: w337 -> [w343 _]
              tunnel: w334 -> [w342 _]
              frame True {
                n130 = invoke class="VI" method="FP.Open"(reference=w343, error in=w344, "State"=w342) -> (error out=w345:errorcluster)  [unwired: 2 in, 4 out]
              }
              frame False {
              }
            }
          }
        }
        n131 = call <vilib>:"Add State(s) to Queue__jki_lib_state_machine.vi"("State(s) in (\"\")"=w281) -> ("States Out"=w280:string)  [unwired: 14 in]
      }
      frame "---------- Macro ----------" {
        # "Do not put any code in this frame.\n(It is a separator no-op. You can make a copy of this frame to create a new Macro frame)"
        n132 = call <vilib>:"Add State(s) to Queue__jki_lib_state_machine.vi"("State(s) in (\"\")"=w351) -> ("States Out"=w350:string)  [unwired: 14 in]
      }
      frame "Macro: Initialize" {
        # "Initialization Macro\n(This is called once, when the VI starts)"
        n133 = call <vilib>:"Add State(s) to Queue__jki_lib_state_machine.vi"("State(s) in Front (\"\")"="Data: Initialize\nInitialize Core Data\nAction: Create and Start Filters\nAction: Load Binaries\nEvents: Register\nUI: Initialize\nUI: Front Panel State >> Open\nAction: Populate Listbox", "State(s) in (\"\")"=w357) -> ("States Out"=w356:string)  [unwired: 13 in]
      }
      frame "Macro: Exit" {
        # "Exit Macro\n(This is called once, when the VI exits)"
        n134 = Unbundle By Name(w365) -> ("Core.Close Panel on Exit?"=w360:bool)
        n135 = call <vilib>:"Conditional State String__jki_lib_state_machine.vi"("Do State(s)?"=w360, "State"="UI: Front Panel State >> Close") -> ("State Out"=w359:string)  [unwired: 7 in]
        n136 = call <vilib>:"Add State(s) to Queue__jki_lib_state_machine.vi"("State(s) in (\"\")"=w359, "State(s) at Back (\"\")"="UI: Uninitialize\nData: Cleanup\nEvents: Unregister\nExit") -> ("States Out"=w363:string)  [unwired: 13 in]
        n137 = call <vilib>:"Add State(s) to Queue__jki_lib_state_machine.vi"("State(s) in Front (\"\")"=w363, "State(s) in (\"\")"=w367) -> ("States Out"=w366:string)  [unwired: 13 in]
      }
      frame "---------- Action ----------" {
        n138 = call <vilib>:"Add State(s) to Queue__jki_lib_state_machine.vi"("State(s) in (\"\")"=w372) -> ("States Out"=w371:string)  [unwired: 14 in]
      }
      frame "Action: Send Filters" {
        n139 = Unbundle By Name(w387) -> ("filters events"=w378:refnum<user-event>, "filters.team filter"=w386:refnum<class "selection_dropdown.lvclass">, "filters.story filter"=w385:refnum<class "selection_dropdown.lvclass">, "filters.char filter"=w384:refnum<class "selection_dropdown.lvclass">, "filters.concept filter"=w383:refnum<class "selection_dropdown.lvclass">)
        n140 = call "Filter List.get.vi"("selection_dropdown in"=w386) -> ("filter list"=w382:string[])  [unwired: 9 in, 1 out]
        n141 = call "Filter List.get.vi"("selection_dropdown in"=w385) -> ("filter list"=w381:string[])  [unwired: 9 in, 1 out]
        n142 = call "Filter List.get.vi"("selection_dropdown in"=w384) -> ("filter list"=w380:string[])  [unwired: 9 in, 1 out]
        n143 = call "Filter List.get.vi"("selection_dropdown in"=w383) -> ("filter list"=w379:string[])  [unwired: 9 in, 1 out]
        n144 = Bundle(cluster=T6 {"team filter"=[], "story filter"=[], "char filter"=[], "concept filter"=[], "Apply Filters"=enum."AND"} ("output cluster"), "team filter"=w382, "story filter"=w381, "char filter"=w380, "concept filter"=w379, "Apply Filters"="Apply Filters") -> (w374:T6)
        n145 = Generate User Event(user event=w378, event data cluster=w374, error in=w377) -> (error out=w376:errorcluster)  [unwired: 1 in, 1 out]
        n146 = call <vilib>:"Add State(s) to Queue__jki_lib_state_machine.vi"("State(s) in (\"\")"=w390) -> ("States Out"=w389:string)  [unwired: 14 in]
      }
      frame "Action: Load Binaries" {
        n147 = in-place {
          in-place-border: w392 -> [w403]
          in-place-border: [w402] -> w391
          n148 = in-place-cluster #5(w394) -> ("manager_daemon"=w401:refnum<class "manager_daemon.lvclass">, "filters"=w399:T8)
          n149 = call "selections.load.binaries.vi"("error in (no error)"=w403, "filters"=w399, "manager_daemon"=w401) -> ("error out"=w402:errorcluster, "filters out"=w398:T8, "manager_daemon out"=w400:refnum<class "manager_daemon.lvclass">)  [unwired: 6 in]
          n150 = in-place-cluster #5("manager_daemon"=w400, "filters"=w398) -> (w393:T7)
        }
        n151 = call <vilib>:"Add State(s) to Queue__jki_lib_state_machine.vi"("State(s) in (\"\")"=w397) -> ("States Out"=w396:string)  [unwired: 14 in]
      }
      frame "Action: Create and Start Filters" {
        n152 = control-ref of="team filter"() -> (w418:refnum<vi>)
        n153 = control-ref of="storyArc filter"() -> (w417:refnum<vi>)
        n154 = control-ref of="character filter"() -> (w416:refnum<vi>)
        n155 = control-ref of="concept filter"() -> (w415:refnum<vi>)
        n156 = call "Create.vi"("error in (no error)"=w414, "ref"=w418) -> ("error out"=w426:errorcluster, "selection_dropdown out"=w425:refnum<class "selection_dropdown.lvclass">)  [unwired: 8 in]
        n157 = call "Create.vi"("error in (no error)"=w414, "ref"=w417) -> ("error out"=w423:errorcluster, "selection_dropdown out"=w424:refnum<class "selection_dropdown.lvclass">)  [unwired: 8 in]
        n158 = call "Create.vi"("error in (no error)"=w414, "ref"=w416) -> ("error out"=w422:errorcluster, "selection_dropdown out"=w421:refnum<class "selection_dropdown.lvclass">)  [unwired: 8 in]
        n159 = call "Create.vi"("error in (no error)"=w414, "ref"=w415) -> ("error out"=w419:errorcluster, "selection_dropdown out"=w420:refnum<class "selection_dropdown.lvclass">)  [unwired: 8 in]
        n160 = call "Start.vi"("error in (no error)"=w426, "selection_dropdown in"=w425) -> ("error out"=w412:errorcluster, "selection_dropdown out"=w413:refnum<class "selection_dropdown.lvclass">)  [unwired: 8 in]
        n161 = call "Start.vi"("error in (no error)"=w423, "selection_dropdown in"=w424) -> ("error out"=w411:errorcluster, "selection_dropdown out"=w407:refnum<class "selection_dropdown.lvclass">)  [unwired: 8 in]
        n162 = call "Start.vi"("error in (no error)"=w422, "selection_dropdown in"=w421) -> ("error out"=w410:errorcluster, "selection_dropdown out"=w406:refnum<class "selection_dropdown.lvclass">)  [unwired: 8 in]
        n163 = call "Start.vi"("error in (no error)"=w419, "selection_dropdown in"=w420) -> ("error out"=w409:errorcluster, "selection_dropdown out"=w405:refnum<class "selection_dropdown.lvclass">)  [unwired: 8 in]
        n164 = flat-sequence {
          tunnel: w412 -> [w435]
          tunnel: w411 -> [w434]
          tunnel: w410 -> [w433]
          tunnel: w409 -> [w432]
          tunnel: [w431] -> w408
          frame #0 {
            # "Allow for startup"
            n165 = Merge Errors(w435, w434, w433, w432) -> (w431:errorcluster)
            n166 = Wait (ms)(milliseconds to wait=u32 100) -> ()  [unwired: 1 out]
          }
        }
        n167 = Bundle By Name(cluster=w427, "filters.team filter"=w413, "filters.story filter"=w407, "filters.char filter"=w406, "filters.concept filter"=w405) -> (w404:T7)
        n168 = call <vilib>:"Add State(s) to Queue__jki_lib_state_machine.vi"("State(s) in (\"\")"=w430) -> ("States Out"=w429:string)  [unwired: 14 in]
      }
      frame "Action: Populate Listbox" {
        # "Your code here.\n(You can make a copy of, or modify, this frame)"
        n169 = for {
          tunnel: "map" -> [w471] mode=indexing
          tunnel: [w466] -> w448 mode=indexing
          tunnel: [w458] -> w447 mode=indexing
          tunnel: [w463] -> w446 mode=indexing
          tunnel: "filtered publisher ids" -> [w464]
          n170 = Unbundle By Name(w471) -> ("value.id"=w463:i32, "name"=w468:string, "value.volumes"=w470:set{i32})
          n171 = Search 1D Array(1D array=w464, element=w463) -> (index of element=w460:i32)  [unwired: 1 in]
          n172 = Collection Size(1:w470) -> (0:w469:i32)
          n173 = Greater Or Equal To 0?(x=w460) -> (x >= 0?=w459:bool)
          n174 = Number To Decimal String(number=w463) -> (decimal integer string=w465:string)  [unwired: 1 in]
          n175 = Number To Decimal String(number=w469) -> (decimal integer string=w467:string)  [unwired: 1 in]
          n176 = Select(t=1, s=w459, f=0) -> (s? t:f=w458:i32)
          n177 = Build Array(w465, w468, w467) -> (w466:string[])
        }
        n178 = Array Size(array=w447) -> (size(s)=w443:i32)
        n179 = Bundle By Name(cluster=w450, "pub ids"=w446, "pub symbols"=w447) -> (w449:T7)
        n180 = In Range and Coerce(upper limit=20, x=w443, lower limit=0) -> (coerced(x)=w440:i32, In Range?=w439:bool)
        n181 = Not(x=w439) -> (.not. x?=w438:bool)
        n182 = property on="pub listbox" class="MCListbox (strict)"(error in=w452, "ColHdrString"=string[] ["ID", "Publisher", "Count"] ("Row Header Strings[]"), "NumCols"=u32 3 ("Number of Columns"), "ItemNames"=w448, "ItemSyms"=w447, "NumRows"=w440, "Value"=-1 ("Multicolumn Listbox"), "VScrollVis"=w438) -> (error out=w451:errorcluster)  [unwired: 1 in, 1 out]
        n183 = call <vilib>:"Add State(s) to Queue__jki_lib_state_machine.vi"("State(s) in (\"\")"=w457) -> ("States Out"=w456:string)  [unwired: 14 in]
      }
      frame "Action: Send Publishers" {
        n184 = Unbundle By Name(w479) -> ("pub ids"=w477:i32[], "pub symbols"=w478:i32[], "pub filter event"=w476:refnum<user-event>)
        n185 = for {
          tunnel: w478 -> [w485] mode=indexing
          tunnel: [w483] -> w473 mode=indexing if=w482
          tunnel: w477 -> [w483] mode=indexing
          n186 = Equal?(x=w485, y=1) -> (x = y?=w482:bool)
        }
        n187 = Generate User Event(user event=w476, event data cluster=w473, error in=w475) -> (error out=w474:errorcluster)  [unwired: 1 in, 1 out]
        n188 = call <vilib>:"Add State(s) to Queue__jki_lib_state_machine.vi"("State(s) in (\"\")"=w481) -> ("States Out"=w480:string)  [unwired: 14 in]
      }
    }
  }
